vi "upload.vi"(8 "error in (no error)":errorcluster, 11 "CameraControlViewer in":refnum<class "CameraControlViewer.lvclass">) -> (0 "error out":errorcluster, 3 "CameraControlViewer out":refnum<class "CameraControlViewer.lvclass">)   [LabVIEW 2011, in "Views.lvlib" / "Camera.lvlib" / "CameraControlViewer.lvclass"]
uses:
  CameraControlViewer.lvclass
  CameraControlViewer.lvclass/CameraControlViewer.ctl
  Tools/Filing/FileSystem/FileSystem.lvclass
  Tools/CameraSettings/CamaraSettings.lvclass
  Tools/Settings.lvlib
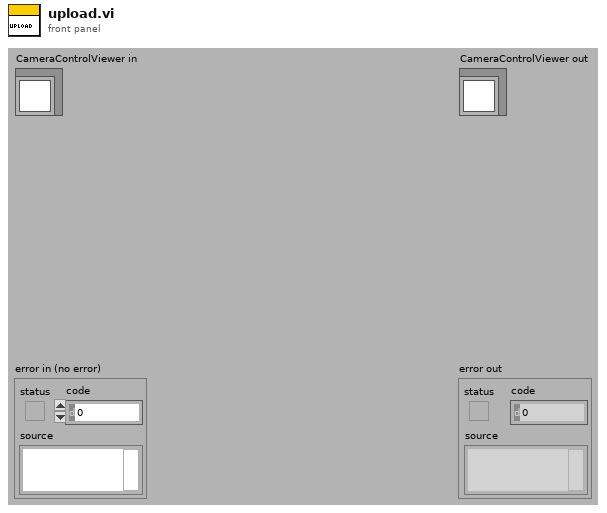
[diagram p1: front panel]
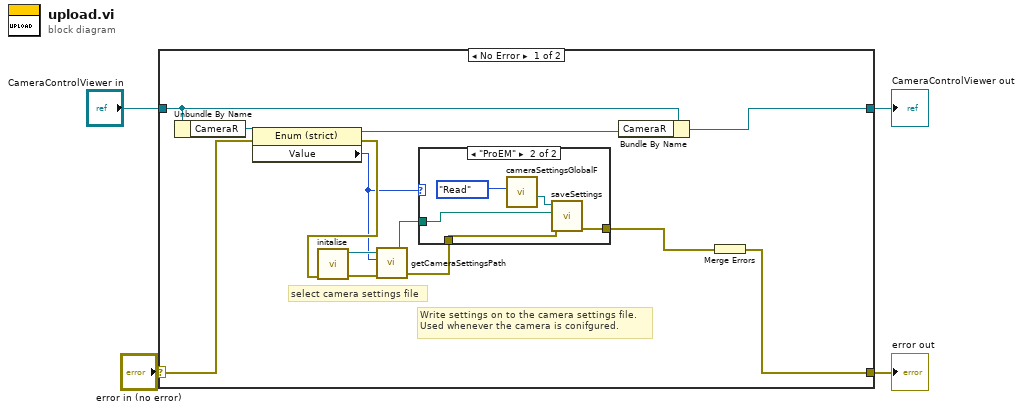
[diagram p0: block diagram]
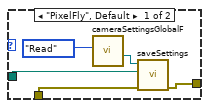
[diagram p2: hidden frame]
diagram:
  n1 = case shown="No Error" "error in (no error)" {
    selector: "error in (no error)" -> [w10 w29]
    tunnel: [w15 w29] -> w3
    tunnel: [w6 w28] -> w1
    tunnel: "CameraControlViewer in" -> [w7 w28]
    frame No Error {
      # "select camera settings file"
      # "Write settings on to the camera settings file.\nUsed whenever the camera is conifgured."
      n2 = Unbundle By Name(w7) -> ("CameraR"=w11:refnum<vi>)
      n3 = property class="Enum (strict)"(reference=w11, error in=w10) -> (reference out=w8:refnum<vi>, error out=w9:errorcluster, "Value"=w5:enum16{"Pixis", "ProEM", "PixelFly"})
      n4 = call "initalise.vi"("error in (no error)"=w9) -> ("error out"=w16:errorcluster, "FileSystem out"=w17:refnum<class "FileSystem.lvclass">)  [unwired: 9 in]
      n5 = call-dynamic "getCameraSettingsPath.vi"("error in (no error)"=w16, "Camera"=w5, "FileSystem.lvclass in"=w17) -> ("error out"=w13:errorcluster, "CameraSettingsPath"=w14:path)  [unwired: 6 in, 1 out]
      n6 = case shown="\"ProEM\"" w5 {
        tunnel: w14 -> [w21 w25]
        tunnel: w13 -> [w19 w24]
        tunnel: [w18 w23] -> w12
        frame "PixelFly", Default {
          n7 = call "cameraSettingsGlobalF.vi"("Action"=enum16{"Write", "Read"}."Read") -> ("CamaraSettings"=w20:refnum<class "CamaraSettings.lvclass">)  [unwired: 10 in]
          n8 = call-dynamic "saveSettings.vi"("error in (no error)"=w19, "Path"=w21, "CamaraSettings in"=w20) -> ("error out"=w18:errorcluster)  [unwired: 7 in, 1 out]
        }
        frame "ProEM" {
          n9 = call "cameraSettingsGlobalF.vi"("Action"=enum16{"Write", "Read"}."Read") -> ("CamaraSettings"=w26:refnum<class "CamaraSettings.lvclass">)  [unwired: 10 in]
          n10 = call-dynamic "saveSettings.vi"("error in (no error)"=w24, "Path"=w25, "CamaraSettings in"=w26) -> ("error out"=w23:errorcluster)  [unwired: 7 in, 1 out]
        }
      }
      n11 = Bundle By Name(cluster=w7, "CameraR"=w8) -> (w6:refnum<class "CameraControlViewer.lvclass">)
      n12 = Merge Errors(w12) -> (w15:errorcluster)
    }
    frame Error {
    }
  }
  "error out" <- w3
  "CameraControlViewer out" <- w1
